vi "Timer FGV.vi"(8 "error in (no error)":errorcluster, 10 "Time target (s)":dbl, 11 "Timer mode":T1(ring)) -> (0 "error out":errorcluster, 1 "Started from reset?":bool, 2 "Time Elapsed?":bool, 3 "Elapsed time (s)":dbl)   [LabVIEW 2025]
doc: "Timer as a functional global variable. The timer mode can be changed globally in the application."
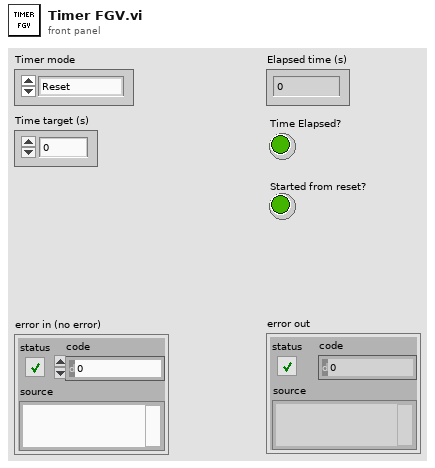
[diagram p1: front panel]
types:
  T1 = enum16{"Reset", "Start", "Read", "Pause", "Resume"}
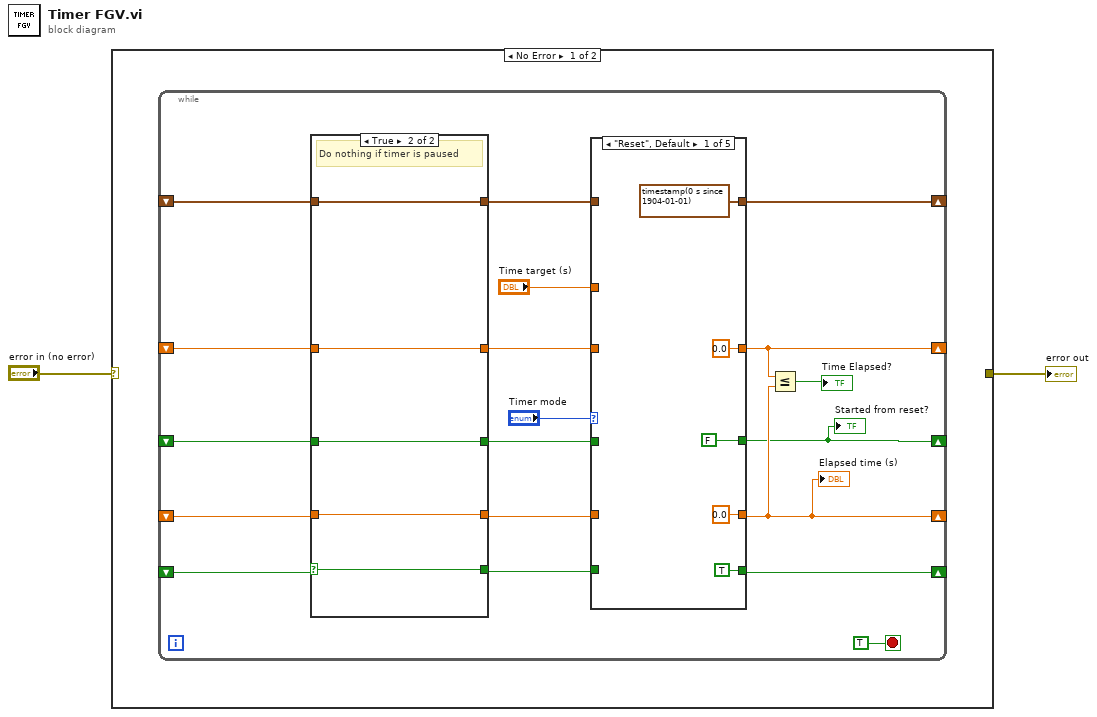
[diagram p0: block diagram]
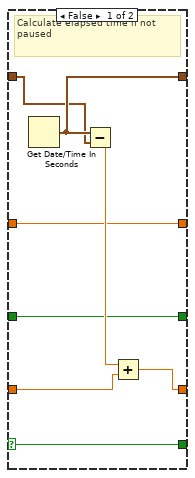
[diagram p2: hidden frame]
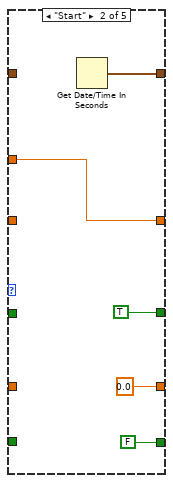
[diagram p3: hidden frame]
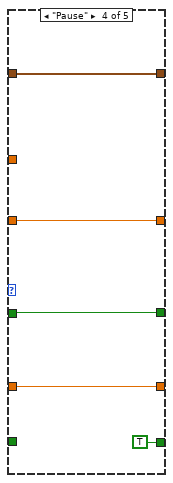
[diagram p5: hidden frame]
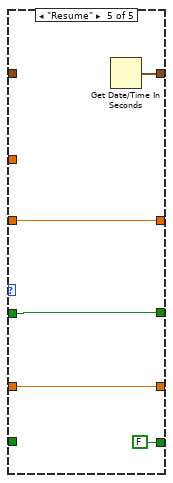
[diagram p6: hidden frame]
diagram:
  n1 = case shown="No Error" "error in (no error)" {
    selector: "error in (no error)" -> [_ w60]
    tunnel: [_ w60] -> w1
    frame No Error {
      n2 = while {
        shift-right: [w8] -> _
        shift-left: _ -> [w13]
        shift-right: [w18] -> _
        shift-left: _ -> [w15]
        shift-right: [w7] -> _
        shift-left: _ -> [w11]
        shift-right: [w17] -> _
        shift-left: _ -> [w16]
        shift-right: [w5] -> _
        shift-left: _ -> [w4]
        stop <- TRUE stop-if-true
        n3 = case shown="True" w16 {
          selector: w16 -> [w23 w31]
          tunnel: w15 -> [w28 w34]
          tunnel: [w29 w34] -> w14
          tunnel: [w24 w33] -> w12
          tunnel: w13 -> [w24 w33]
          tunnel: [w25 w32] -> w10
          tunnel: w11 -> [w27 w32]
          tunnel: [w23 w31] -> w9
          tunnel: w4 -> [w22 w30]
          tunnel: [w22 w30] -> w3
          frame False {
            # "Calculate elapsed time if not paused"
            n4 = Get Date/Time In Seconds() -> (seconds since 1Jan1904=w29:timestamp)
            n5 = Subtract(x=w29, y=w28) -> (x-y=w26:dbl)
            n6 = Add(x=w26, y=w27) -> (x+y=w25:dbl)
          }
          frame True {
            # "Do nothing if timer is paused"
          }
        }
        n7 = case shown="\"Reset\", Default" "Timer mode" {
          tunnel: "Time target (s)" -> [_ w44 _ _ _]
          tunnel: [0.0 ("Time target (s)") w44 w48 w53 w59] -> w8
          tunnel: [timestamp(0 s since 1904-01-01) ("seconds since 1Jan1904") w43 w49 w54 w56] -> w18
          tunnel: [0.0 0.0 w47 w52 w58] -> w7
          tunnel: [TRUE FALSE w46 TRUE FALSE] -> w17
          tunnel: w14 -> [_ _ w49 w54 _]
          tunnel: w12 -> [_ _ w48 w53 w59]
          tunnel: w10 -> [_ _ w47 w52 w58]
          tunnel: w9 -> [_ _ w46 _ _]
          tunnel: [FALSE TRUE w45 w50 w55] -> w5
          tunnel: w3 -> [_ _ w45 w50 w55]
          frame "Reset", Default {
          }
          frame "Start" {
            n8 = Get Date/Time In Seconds() -> (seconds since 1Jan1904=w43:timestamp)
          }
          frame "Read" {
          }
          frame "Pause" {
          }
          frame "Resume" {
            n9 = Get Date/Time In Seconds() -> (seconds since 1Jan1904=w56:timestamp)
          }
        }
        "Elapsed time (s)" <- w7
        "Started from reset?" <- w5
        n10 = Less Or Equal?(x=w8, y=w7) -> (x <= y?=→"Time Elapsed?":bool)
      }
    }
    frame Error {
    }
  }
  "error out" <- w1
